vi "Filter_Set focus.vi"(11 "Fillter String Ref":refnum<vi>) -> (3 "Fillter String Ref out":refnum<vi>)   [LabVIEW 2023]
doc: "Set focus on filter and select text is filter test entry exists."
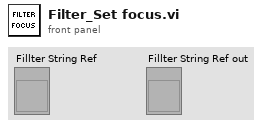
[diagram p1: front panel]
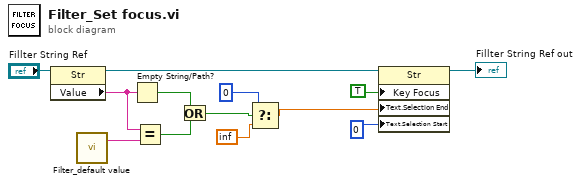
[diagram p0: block diagram]
diagram:
  n1 = property class="Str"(reference="Fillter String Ref") -> (reference out=w10:refnum<vi>, "Value"=w9:string)  [unwired: 1 in, 1 out]
  n2 = call "Filter_default value.vi"() -> ("Filter Default Value"=w8:string)  [unwired: 3 in]
  n3 = Empty String/Path?(string/path=w9) -> (empty?=w7:bool)
  n4 = Equal?(x=w9, y=w8) -> (x = y?=w6:bool)
  n5 = Or(x=w7, y=w6) -> (x .or. y?=w5:bool)
  n6 = Select(t=u32 0 ("Text.Selection:Start"), s=w5, f=inf) -> (s? t:f=w2:dbl)
  n7 = property class="Str"(reference=w10, "Key Focus"=TRUE, "Text.Selection End"=w2, "Text.Selection Start"=u32 0 ("Text.Selection:Start")) -> (reference out=→"Fillter String Ref out":refnum<vi>)  [unwired: 1 in, 1 out]
